vi "SMTP Email Send Data.vi"(0 "recipients":string[](array[string]), 1 "mail server":string, 2 "return address":string, 5 "subject ([No Subject])":string="[No Subject]", 7 "message":string, 9 "data":string, 11 "error in (no error)":errorcluster, 12 "binary? (F)":bool, 13 "MIME content-type (application/octet-stream)":string="application/octet-stream") -> (4 "invalid recipients":string[](array[string]), 15 "error out":errorcluster)   [LabVIEW 2011, in "NewNI_SMTPEmail.lvlib"]
doc: "Sends an email with attached data to a list of recipients."
uses:
  NewNI_SMTPEmail.lvlib
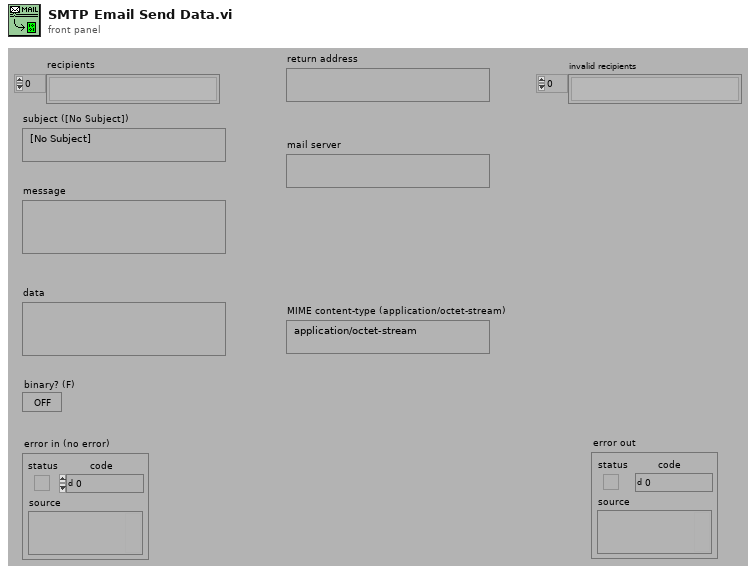
[diagram p1: front panel]
types:
  T1 = cluster{path, "data":string, "binary? (F)":bool, "MIME content-type (application/octet-stream)":string}
  T2 = cluster{path, "data":string, "binary? (F)":bool, "MIME content-type (application/octet-stream)":string}[]
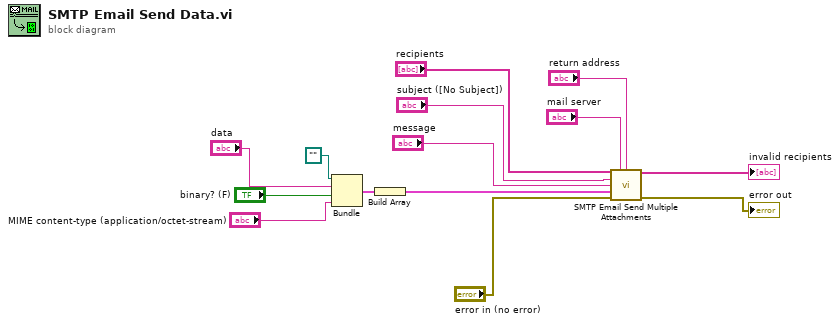
[diagram p0: block diagram]
diagram:
  n1 = Bundle(path "", "data"="data", "binary? (F)"="binary? (F)", "MIME content-type (application/octet-stream)"="MIME content-type (application/octet-stream)") -> (w3:T1)  [unwired: 1 out]
  n2 = Build Array(w3) -> (w2:T2)
  n3 = call "SMTP Email Send Multiple Attachments.vi"("recipients"="recipients", "mail server"="mail server", "return address"="return address", "subject ([No Subject])"="subject ([No Subject])", "message"="message", "attachments"=w2, "error in (no error)"="error in (no error)") -> ("invalid recipients"=→"invalid recipients":string[], "error out"=→"error out":errorcluster)  [unwired: 1 in, 6 out]
